vi "Calcu_Weight.vi"(4 "Measured":string[][](array[string]), 6 "공기밀도":string, 8 "측정횟수":i32, 10 "분해능자리수":i32, 11 "분동식별표기":string[][](array[string])) -> (1 "X=S-T":string[][](array[string]), 3 "분동식별표기":string[][](array[string]))   [LabVIEW 2020]
uses:
  <vilib>/express/express arith-compare/Formula/XNode/ExpressFormulaBlockNode.xnode
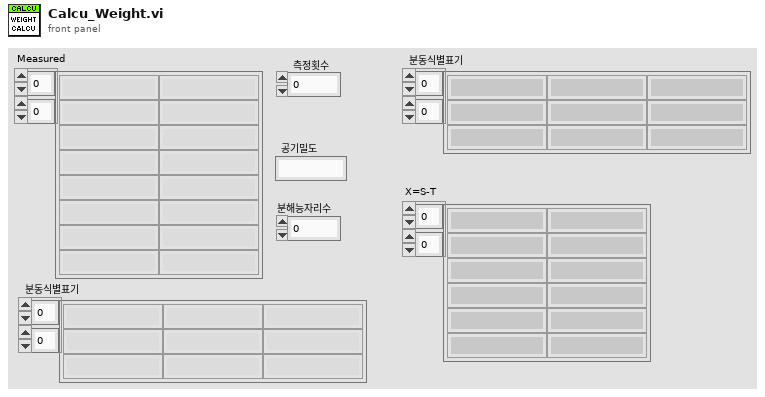
[diagram p1: front panel]
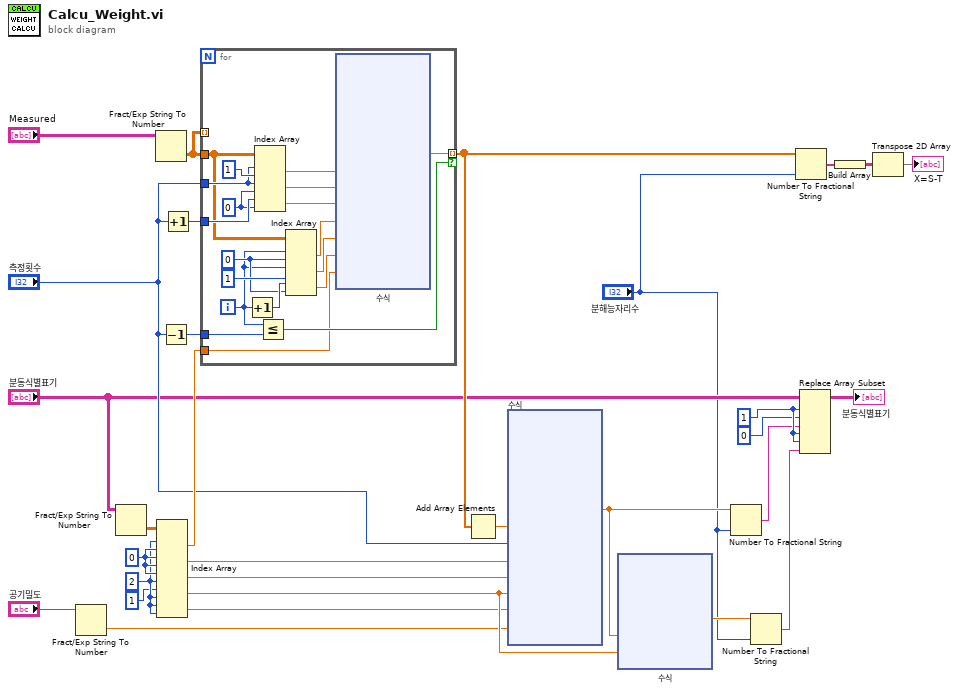
[diagram p0: block diagram]
diagram:
  w29 = 1 ("인덱스 (행)")
  w16 = 2 ("비활성화된 인덱스 (열)")
  w17 = 0 ("인덱스 (행)")
  n1 = Fract/Exp String To Number(string="공기밀도") -> (number=w12:dbl)  [unwired: 3 in, 1 out]
  n2 = Fract/Exp String To Number(string="분동식별표기") -> (number=w9:dbl[][])  [unwired: 3 in, 1 out]
  n3 = Fract/Exp String To Number(string="Measured") -> (number=w5:dbl[][])  [unwired: 3 in, 1 out]
  n4 = Index Array(array=w9, index (row) #1=w16, index (col) #1=w17, index (row) #2=w17, index (col) #2=w17, index (row) #3=w17, index (col) #3=w16, index (row) #4=1 ("인덱스 (행)"), index (col) #4=w16, index (row) #5=w16, index (col) #5=w16) -> (element #1=w18:dbl, element #2=w10:dbl, element #3=w13:dbl, element #4=w27:dbl, element #5=w15:dbl)
  n5 = Decrement(x="측정횟수") -> (x-1=w3:i32)
  n6 = Increment(x="측정횟수") -> (x+1=w6:i32)
  n7 = for {
    tunnel: w5 -> [_] mode=indexing
    tunnel: w18 -> [w38]
    tunnel: w6 -> [w47]
    tunnel: w5 -> [w45]
    tunnel: "측정횟수" -> [w48]
    tunnel: [w31] -> w8 mode=indexing if=w39
    tunnel: w3 -> [w41]
    i -> [w40]
    w42 = 0 ("비활성화된 인덱스 (열)")
    w46 = 0 ("비활성화된 인덱스 (열)")
    n8 = Increment(x=w40) -> (x+1=w43:i32)
    n9 = Index Array(array=w45, index (row) #1=w48, index (col) #1=1 ("비활성화된 인덱스 (열)"), index (row) #2=w48, index (col) #2=w46, index (row) #3=w47, index (col) #3=w46) -> (element #1=w32:dbl, element #2=w37:dbl, element #3=w36:dbl)
    n10 = Less Or Equal?(x=w40, y=w41) -> (x <= y?=w39:bool)
    n11 = Index Array(array=w45, index (row) #1=w40, index (col) #1=w42, index (row) #2=w40, index (col) #2=1 ("비활성화된 인덱스 (열)"), index (row) #3=w43, index (col) #3=w42) -> (element #1=w35:dbl, element #2=w34:dbl, element #3=w33:dbl)
    n12 = xnode "수식"("O22"=w32, "O21"=w37, "O23"=w36, "Oi"=w35, "Oi1"=w34, "Oi2"=w33, "Δms"=w38) -> ("결과"=w31:dbl)  [unwired: 1 in, 1 out]
  }
  n13 = Add Array Elements(numeric array=w8) -> (sum=w19:dbl)
  n14 = xnode "수식"("Dmx"=w19, "X"="측정횟수", "Ms"=w10, "dS"=w13, "dT"=w27, "dDms"=w15, "ro"=w12) -> ("결과"=w26:dbl)  [unwired: 1 in, 1 out]
  n15 = xnode "수식"("Mt"=w26, "dT"=w27) -> ("결과"=w28:dbl)  [unwired: 1 in, 1 out]
  n16 = Number To Fractional String(number=w26, precision (6)="분해능자리수") -> (F-format string=w22:string)  [unwired: 2 in]
  n17 = Number To Fractional String(number=w28, precision (6)="분해능자리수") -> (F-format string=w30:string)  [unwired: 2 in]
  n18 = Number To Fractional String(number=w8, precision (6)="분해능자리수") -> (F-format string=w23:string[])  [unwired: 2 in]
  n19 = Replace Array Subset(array="분동식별표기", new element #1=w22, index (row) #1=w29, index (col) #1=0 ("비활성화된 인덱스 (열)"), new element #2=w30, index (row) #2=w29, index (col) #2=w29) -> (→"분동식별표기":string[][])
  n20 = Build Array(w23) -> (w24:string[][])
  n21 = Transpose 2D Array(2D array=w24) -> (transposed array=→"X=S-T":string[][])
